vi "sub_calc-potential-field.vi"(6 "start pt":cluster{"x":dbl, "y":dbl}, 10 "obstacles":cluster{"x":dbl, "y":dbl}[](array[cluster]), 11 "goal pt":cluster{"x":dbl, "y":dbl}) -> (2 "minxy":cluster{dbl, dbl}, 3 "pmap":T1)   [LabVIEW 2019]
uses:
  <vilib>/Analysis/Matrix/Datatypes/RealMatrix.ctl
  Ctrl/cmd_common.ctl
  <vilib>/Analysis/Matrix/Numeric/Conversions/Array To Matrix - RA2.vi
  <vilib>/Analysis/Matrix/NI_Matrix.lvlib
panel:
  out "Intensity Graph":dbl[][](graph)
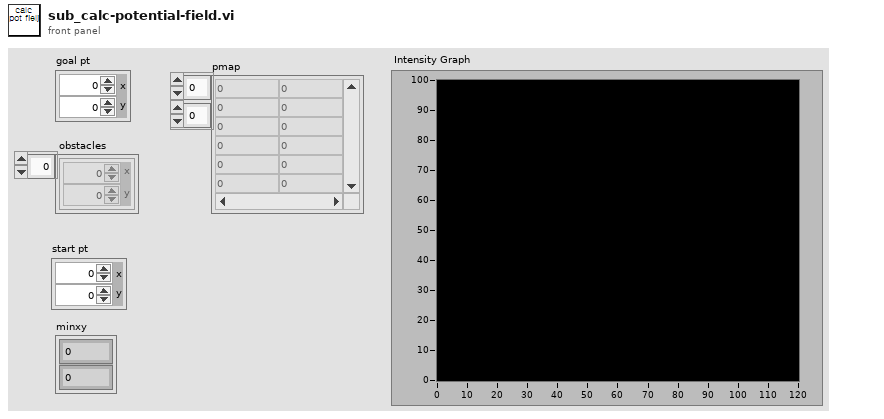
[diagram p1: front panel]
types:
  T1 = typedef "NI_Matrix.lvlib/RealMatrix.ctl" = dbl[][]
  T2 = typedef "cmd_common.ctl" = enum16{"read", "write"}
  T3 = cluster{"KP":dbl, "ETA":dbl, "AREA_WIDTH":dbl, "Osc_Det_Len":u32}
  T4 = cluster{"start pt":cluster{"x":i32, "y":dbl}, "goal pt":cluster{"x":i32, "y":i32}, "grid size":dbl, "robot radius":dbl, "obstacles":cluster{"x":i32, "y":i32}[]}
  T5 = cluster{"delay":dbl, "d":dbl, "rxy":cluster{"x":dbl, "y":dbl}[], "pmap":T1}
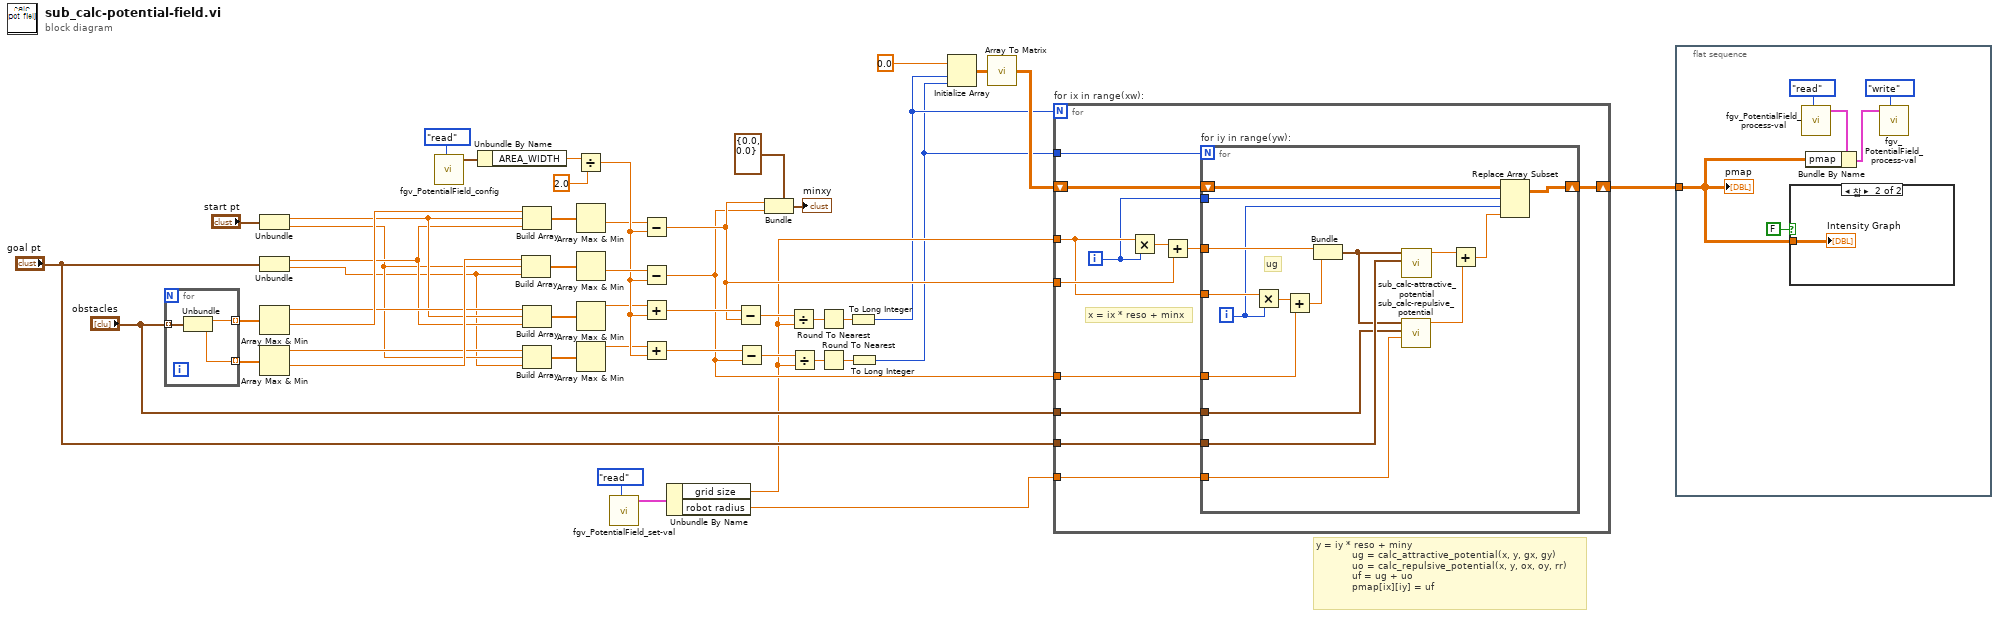
[diagram p0: block diagram]
diagram:
  # "y = iy * reso + miny\n            ug = calc_attractive_potential(x, y, gx, gy)\n            uo = calc_repulsive_potential(x, y, ox, oy, rr)\n            uf = ug + uo\n            pmap[ix][iy] = uf"
  n1 = for {
    tunnel: "obstacles" -> [w51] mode=indexing
    tunnel: [w50] -> w48 mode=indexing
    tunnel: [w49] -> w47 mode=indexing
    n2 = Unbundle(w51) -> ("x"=w50:dbl, "y"=w49:dbl)
  }
  n3 = Unbundle("start pt") -> ("x"=w28:dbl, "y"=w25:dbl)
  n4 = Unbundle("goal pt") -> ("x"=w27:dbl, "y"=w24:dbl)
  n5 = Array Max & Min(array=w48) -> (max value=w29:dbl, min value=w31:dbl)  [unwired: 2 out]
  n6 = Array Max & Min(array=w47) -> (max value=w26:dbl, min value=w32:dbl)  [unwired: 2 out]
  n7 = call "fgv_PotentialField_config.vi"("cmd"=cmd_common."read") -> ("pf-val out"=w43:T3)  [unwired: 10 in]
  n8 = Unbundle By Name(w43) -> ("AREA_WIDTH"=w42:dbl)
  n9 = Build Array(w32, w25, w24) -> (w34:dbl[])
  n10 = Build Array(w31, w28, w27) -> (w45:dbl[])
  n11 = Build Array(w29, w28, w27) -> (w33:dbl[])
  n12 = Build Array(w26, w25, w24) -> (w40:dbl[])
  n13 = Divide(x=w42, y=2.0) -> (x/y=w23:dbl)
  n14 = Array Max & Min(array=w45) -> (min value=w22:dbl)  [unwired: 3 out]
  n15 = Array Max & Min(array=w34) -> (min value=w30:dbl)  [unwired: 3 out]
  n16 = Array Max & Min(array=w33) -> (max value=w21:dbl)  [unwired: 3 out]
  n17 = Array Max & Min(array=w40) -> (max value=w20:dbl)  [unwired: 3 out]
  n18 = call "fgv_PotentialField_set-val.vi"("cmd"=cmd_common."read") -> ("set-val out"=w6:T4)  [unwired: 10 in]
  n19 = Subtract(x=w22, y=w23) -> (x-y=w11:dbl)
  n20 = Subtract(x=w30, y=w23) -> (x-y=w10:dbl)
  n21 = Add(x=w21, y=w23) -> (x+y=w19:dbl)
  n22 = Add(x=w20, y=w23) -> (x+y=w17:dbl)
  n23 = Unbundle By Name(w6) -> ("grid size"=w5:dbl, "robot radius"=w4:dbl)
  n24 = Subtract(x=w19, y=w11) -> (x-y=w38:dbl)
  n25 = Subtract(x=w17, y=w10) -> (x-y=w39:dbl)
  n26 = Bundle(cluster=cluster{"x":dbl, "y":dbl} {"x"=0.0, "y"=0.0} ("start pt"), "x"=w11, "y"=w10) -> (→"minxy":cluster{"x":dbl, "y":dbl})
  n27 = Divide(x=w38, y=w5) -> (x/y=w36:dbl)
  n28 = Divide(x=w39, y=w5) -> (x/y=w37:dbl)
  n29 = Round To Nearest(number=w36) -> (nearest integer value=w18:dbl)
  n30 = Round To Nearest(number=w37) -> (nearest integer value=w16:dbl)
  n31 = To Long Integer(number=w18) -> (32bit integer=w2:i32)
  n32 = To Long Integer(number=w16) -> (32bit integer=w1:i32)
  n33 = Initialize Array(0.0 ("element"), w2, w1) -> (w15:dbl[][])
  n34 = call-poly <vilib>:"Array To Matrix.vi"("Real 2D Array"=w15) -> ("Real Matrix"=w12:T1)
  n35 = for "for ix in range(xw):" {
    N: w2 -> [_]
    tunnel: w1 -> [w63]
    tunnel: w5 -> [w59]
    tunnel: w11 -> [w61]
    tunnel: w10 -> [w58]
    tunnel: "goal pt" -> [w57]
    tunnel: w4 -> [w56]
    tunnel: "obstacles" -> [w55]
    shift-right: [w52] -> w3
    shift-left: w12 -> [w54]
    i -> [w53]
    # "x = ix * reso + minx"
    # "x = ix * reso + minx"
    n36 = Multiply(x=w59, y=w53) -> (x*y=w62:dbl)
    n37 = Add(x=w62, y=w61) -> (x+y=w60:dbl)
    n38 = for "for iy in range(yw):" {
      N: w63 -> [_]
      tunnel: w60 -> [w75]
      tunnel: w59 -> [w79]
      tunnel: w58 -> [w77]
      tunnel: w57 -> [w74]
      tunnel: w56 -> [w72]
      tunnel: w55 -> [w71]
      shift-right: [w64] -> w52
      shift-left: w54 -> [w68]
      tunnel: w53 -> [w67]
      i -> [w66]
      # "ug"
      n39 = Multiply(x=w79, y=w66) -> (x*y=w78:dbl)
      n40 = Add(x=w78, y=w77) -> (x+y=w76:dbl)
      n41 = Bundle(w75, w76) -> (w73:cluster{dbl, dbl})  [unwired: 1 in]
      n42 = call "sub_calc-repulsive_potential.vi"("rr"=w72, "obstacles"=w71, "xy pt"=w73) -> ("return"=w69:dbl)  [unwired: 8 in]
      n43 = call "sub_calc-attractive_potential.vi"("goal pt"=w74, "xy pt"=w73) -> ("length"=w70:dbl)  [unwired: 9 in]
      n44 = Add(x=w70, y=w69) -> (x+y=w65:dbl)
      n45 = Replace Array Subset(array=w68, new element=w65, index (row)=w67, index (col)=w66) -> (w64:T1)
    }
  }
  n46 = flat-sequence {
    tunnel: w3 -> [w80]
    frame #0 {
      n47 = case shown="참" FALSE {
        tunnel: w80 -> [_ w86]
        frame False {
        }
        frame True {
          "Intensity Graph" <- w86
        }
      }
      n48 = call "fgv_PotentialField_process-val.vi"("cmd"=cmd_common."read") -> ("prcess val out"=w82:T5)  [unwired: 10 in]
      n49 = Bundle By Name(cluster=w82, "pmap"=w80) -> (w81:T5)
      n50 = call "fgv_PotentialField_process-val.vi"("cmd"=cmd_common."write", "prcess val"=w81) -> ()  [unwired: 9 in, 1 out]
      "pmap" <- w80
    }
  }
